vi "Check if File or Folder Exists.vi"(8 "error in (no error)":errorcluster, 11 "path":path) -> (0 "error out":errorcluster, 2 "file or folder exists?":bool, 3 "dup path":path)   [LabVIEW 2026]
doc: "<p>Checks whether a file or folder exists on disk at a specified path. This VI works with standard files and folders as well as files in LLB files.</p>"
uses:
  FT_FileTypes.ctl
  NI_FileType.lvlib
  NI_PackedLibraryUtility.lvlib
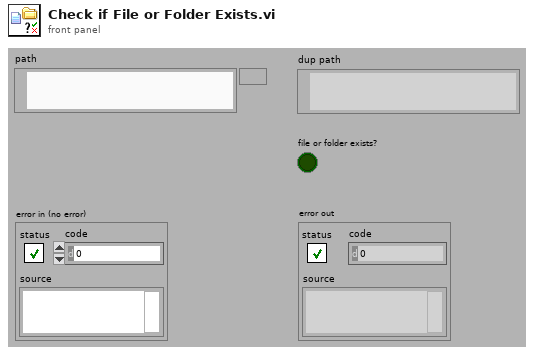
[diagram p1: front panel]
types:
  T1 = typedef "NI_FileType.lvlib/FT_FileTypes.ctl" = enum32{"Invalid file/path", "Unknown type", "Instrument", "Control", "Polymorphic VI", "Project", "Library", "LVClass", "XControl", "XNode", "CIN", "Run-time menu", "Palette menu", "LLB", "Shortcut", "Directory", "Class Private Data Control", "Statechart", "MathScript .m file", "Ladder Diagram", "LVLibp"}
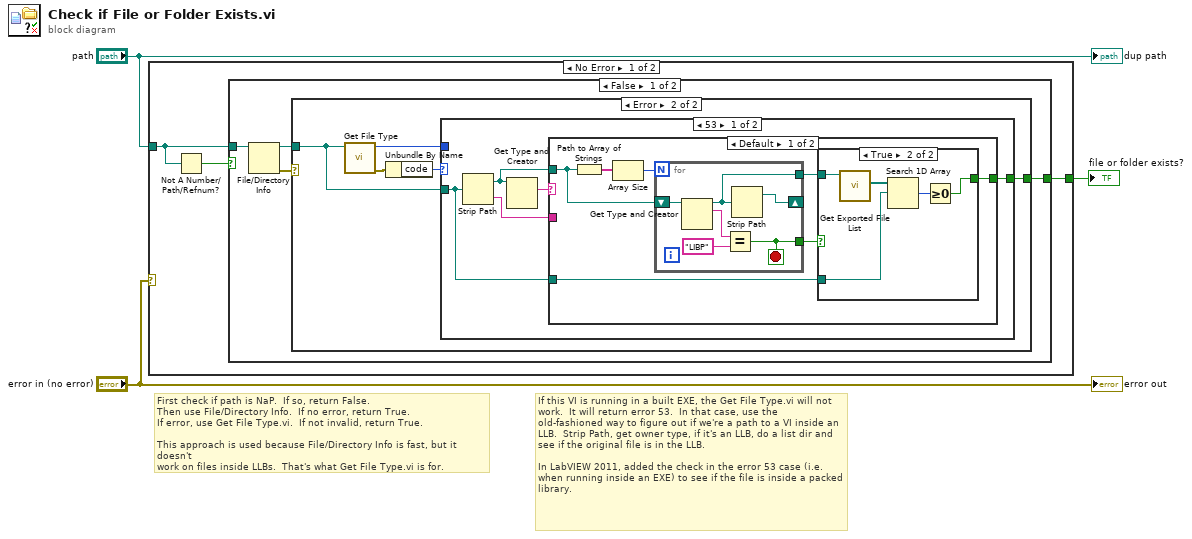
[diagram p0: block diagram]
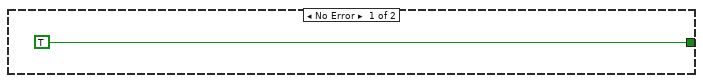
[diagram p2: hidden frame]
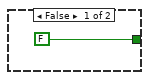
[diagram p3: hidden frame]
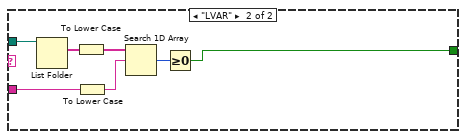
[diagram p4: hidden frame]
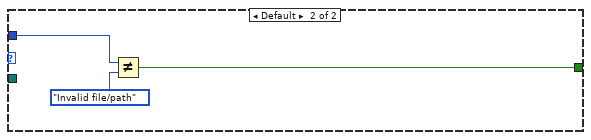
[diagram p5: hidden frame]
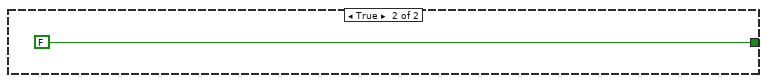
[diagram p6: hidden frame]
diagram:
  # "If this VI is running in a built EXE, the Get File Type.vi will not work.  It will return error 53.  In that case, use the old-fashioned way to figure out if we're a path to a VI inside an LLB.  Strip Path, get owner type, if it's an LLB, do a list dir and see if the original file is in the LLB.\n\nIn LabVIEW 2011, added the check in the error 53 case (i.e. when running inside an EXE) to see if the file is inside a packed library."
  # "First check if path is NaP.  If so, return False.\nThen use File/Directory Info.  If no error, return True.\nIf error, use Get File Type.vi.  If not invalid, return True.\n\nThis approach is used because File/Directory Info is fast, but it doesn't\nwork on files inside LLBs.  That's what Get File Type.vi is for."
  n1 = case shown="No Error" "error in (no error)" {
    tunnel: "path" -> [w5 _]
    tunnel: [w6 _] -> w1
    frame No Error {
      n2 = Not A Number/Path/Refnum?(number/path/refnum=w5) -> (NaN/Path/Refnum?=w4:bool)
      n3 = case shown="False" w4 {
        tunnel: [w8 FALSE] -> w6
        tunnel: w5 -> [w10 _]
        frame False {
          n4 = File/Directory Info(path=w10) -> (path out=w7:path, error out=w9:errorcluster)  [unwired: 1 in, 5 out]
          n5 = case shown="Error" w9 {
            tunnel: [TRUE w16] -> w8
            tunnel: w7 -> [_ w12]
            frame No Error {
            }
            frame Error {
              n6 = call "Get File Type.vi"("path"=w12) -> ("error out"=w14:errorcluster, "file type"=w15:T1)  [unwired: 1 in, 8 out]
              n7 = Unbundle By Name(w14) -> ("code"=w13:i32)
              n8 = case shown="53" w13 {
                tunnel: [w20 w50] -> w16
                tunnel: w15 -> [_ w49]
                tunnel: w12 -> [w17 _]
                frame 53 {
                  n9 = Strip Path(path=w17) -> (stripped path=w18:path, name=w19:string)
                  n10 = Get Type and Creator(7:w18) -> (2:w21:string)  [unwired: 1 in, 3 out]
                  n11 = case shown="Default" w21 {
                    tunnel: [w24 w41] -> w20
                    tunnel: w19 -> [_ w45]
                    tunnel: w18 -> [w26 w47]
                    tunnel: w17 -> [w22 _]
                    frame Default {
                      n12 = Path to Array of Strings(0:w26) -> (2:w28:string[])  [unwired: 1 out]
                      n13 = Array Size(array=w28) -> (size(s)=w27:i32)
                      n14 = for {
                        N: w27 -> [_]
                        shift-right: [w39] -> _
                        shift-left: w26 -> [w40]
                        tunnel: [w36] -> w25
                        tunnel: [w35] -> w23
                        stop <- w36 stop-if-true
                        n15 = Get Type and Creator(7:w40) -> (2:w38:string, 3:w35:path)  [unwired: 1 in, 2 out]
                        n16 = Equal?(x=w38, y="LIBP") -> (x = y?=w36:bool)
                        n17 = Strip Path(path=w35) -> (stripped path=w39:path)  [unwired: 1 out]
                      }
                      n18 = case shown="True" w25 {
                        tunnel: [FALSE w30] -> w24
                        tunnel: w23 -> [_ w34]
                        tunnel: w22 -> [_ w32]
                        frame False {
                        }
                        frame True {
                          n19 = call "Get Exported File List.vi"("packed library path"=w34) -> ("paths"=w33:path[])  [unwired: 8 in, 2 out]
                          n20 = Search 1D Array(1D array=w33, element=w32) -> (index of element=w31:i32)  [unwired: 1 in]
                          n21 = Greater Or Equal To 0?(x=w31) -> (x >= 0?=w30:bool)
                        }
                      }
                    }
                    frame "LVAR" {
                      n22 = List Folder(path=w47) -> (filenames=w46:string[])  [unwired: 1 in, 5 out]
                      n23 = To Lower Case(string=w46) -> (all lower case string=w43:string[])
                      n24 = To Lower Case(string=w45) -> (all lower case string=w44:string)
                      n25 = Search 1D Array(1D array=w43, element=w44) -> (index of element=w42:i32)  [unwired: 1 out]
                      n26 = Greater Or Equal To 0?(x=w42) -> (x >= 0?=w41:bool)
                    }
                  }
                }
                frame Default {
                  n27 = Not Equal?(x=w49, y=FT_FileTypes."Invalid file/path") -> (x != y?=w50:bool)
                }
              }
            }
          }
        }
        frame True {
        }
      }
    }
    frame Error {
    }
  }
  "file or folder exists?" <- w1
  "error out" <- "error in (no error)"
  "dup path" <- "path"
